vi "MT Detect MSK.vi"(5 "input complex waveform":T3={"t0"=0.0, "dt"=1.0, "Y"=[]} {"Y" format="%.3f"; "dt" format="%^.2e"; "t0" format="%.4f"}, 7 "MSK system parameters":T2={"differential encoding enable"=enum."enable", "samples per symbol (16)"=16}, 9 "synchronization parameters":T1 {"sync sequence" format="%.2f"}, 11 "error in (no error)":errorcluster, 12 "matched filter coefficients":dbl[](array[numeric]) format="%.2f", 13 "reset? (T)":bool=TRUE, 14 "flush buffers? (F)":bool) -> (6 "output bit stream":i8[](array[numeric]), 10 "sync found index (symbols)":dbl format="%.4f", 15 "error out":errorcluster)   [LabVIEW 2020, in "niDMT.lvlib"]
doc: "Demodulates an minimum-shift keying (MSK)-modulated complex baseband waveform and returns the demodulated bit stream. This VI attempts to remove carrier and phase offset by locking to the carrier signal."
uses:
  <vilib>/addons/Modulation/niDMT.lvlib
  <vilib>/addons/Modulation/Analog/controls/Complex Data Waveform.ctl
  <vilib>/Utility/error.llb/Error Cluster From Error Code.vi
  <vilib>/addons/Modulation/Digital/Support/Common/mod_Truncate FIR Filter (real).vi
  <vilib>/addons/Modulation/niAMT.lvlib
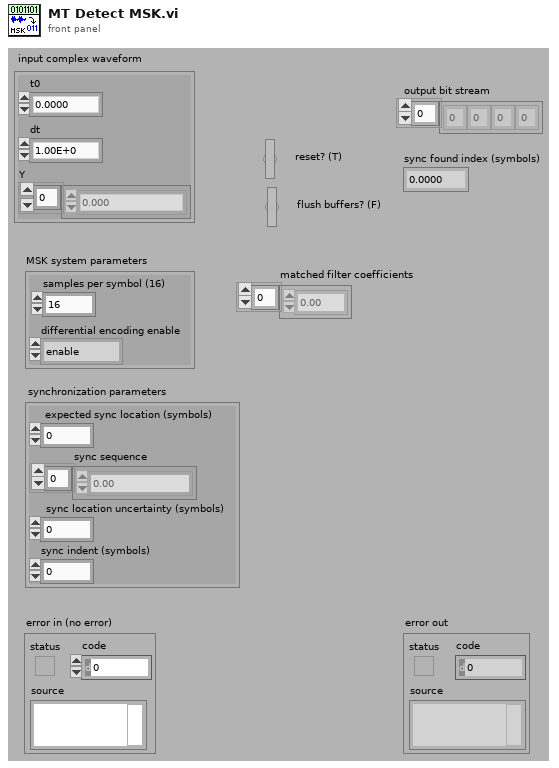
[diagram p1: front panel]
types:
  T1 = cluster{"expected sync location (symbols)":i32, "sync sequence":cdb[], "sync location uncertainty (symbols)":i32, "sync indent (symbols)":i32}
  T2 = cluster{"differential encoding enable":enum16{"disable", "enable"}, "samples per symbol (16)":i32}
  T3 = typedef "niAMT.lvlib/Complex Data Waveform.ctl" = cluster{"t0":dbl, "dt":dbl, "Y":cdb[]}
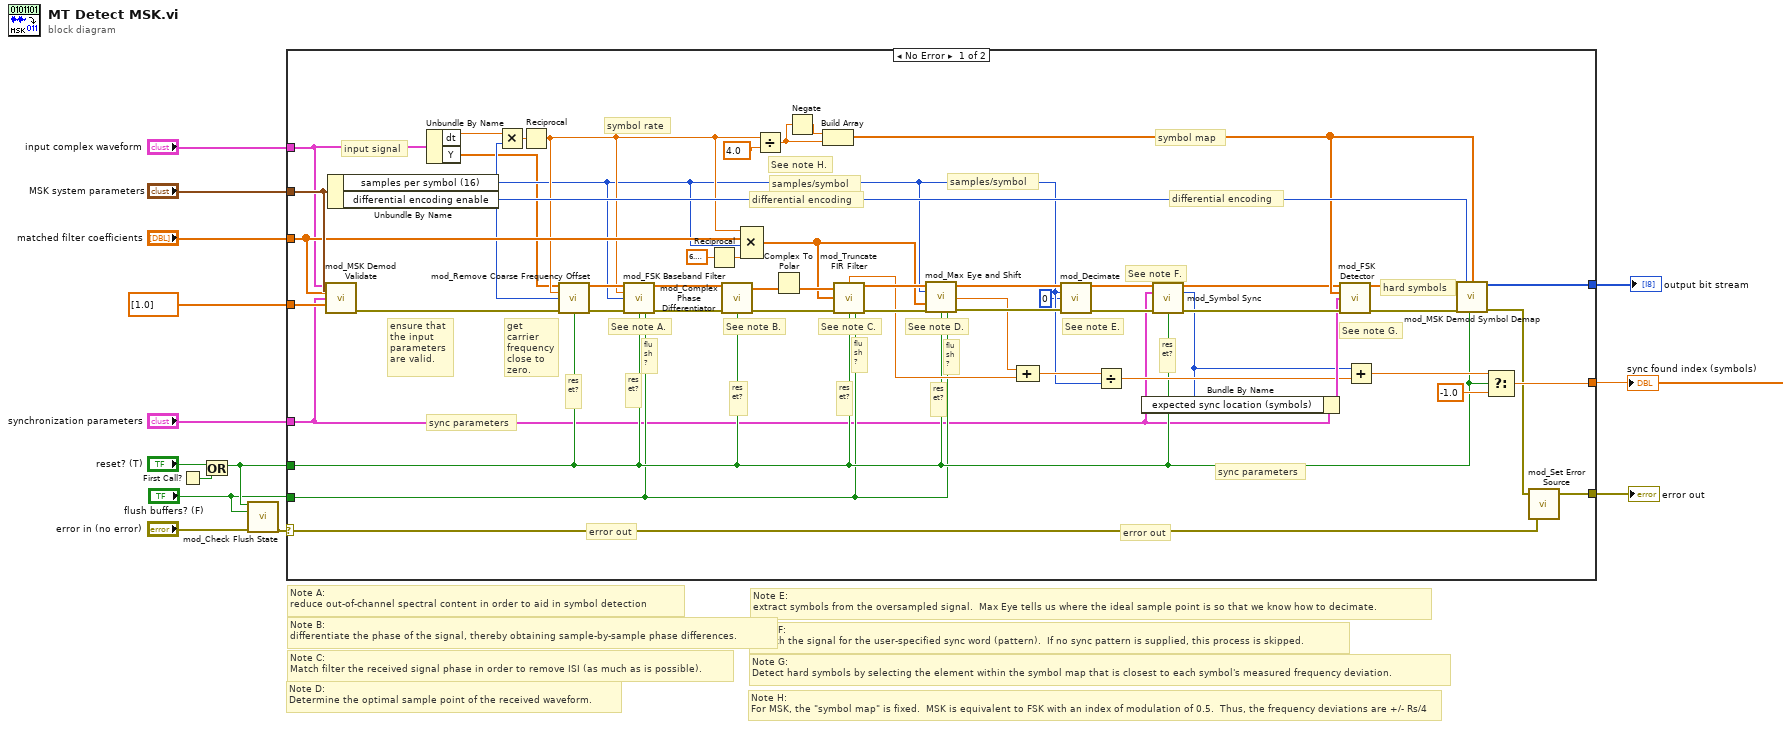
[diagram p0: block diagram]
diagram:
  # "Note H:\nFor MSK, the \"symbol map\" is fixed.  MSK is equivalent to FSK with an index of modulation of 0.5.  Thus, the frequency deviations are +/- Rs/4"
  # "Note A:\nreduce out-of-channel spectral content in order to aid in symbol detection"
  # "Note B:\ndifferentiate the phase of the signal, thereby obtaining sample-by-sample phase differences."
  # "Note C:\nMatch filter the received signal phase in order to remove ISI (as much as is possible)."
  # "Note D:\nDetermine the optimal sample point of the received waveform."
  # "Note E:\nextract symbols from the oversampled signal.  Max Eye tells us where the ideal sample point is so that we know how to decimate."
  # "Note F:\nSearch the signal for the user-specified sync word (pattern).  If no sync pattern is supplied, this process is skipped."
  # "Note G:\nDetect hard symbols by selecting the element within the symbol map that is closest to each symbol's measured frequency deviation."
  n1 = First Call?() -> (First Call?: T/F=w7:bool)
  n2 = Or(x="reset? (T)", y=w7) -> (x .or. y?=w3:bool)
  n3 = call <vilib>:"mod_Check Flush State.vi"("reset?"=w3, "flush buffers? (F)"="flush buffers? (F)", "error in (no error)"="error in (no error)") -> ("error out"=w4:errorcluster)  [unwired: 12 out]
  n4 = case shown="No Error" w4 {
    selector: w4 -> [w54 w67]
    tunnel: [w55 w67] -> w8
    tunnel: "synchronization parameters" -> [w15 _]
    tunnel: "matched filter coefficients" -> [w47 _]
    tunnel: "MSK system parameters" -> [w48 _]
    tunnel: dbl[] [1.0] ("pulse shaping filter coefficients") -> [w46 _]
    tunnel: [w33 _] -> w9
    tunnel: "input complex waveform" -> [w42 _]
    tunnel: [w60 _] -> w10
    tunnel: w3 -> [w27 _]
    tunnel: "flush buffers? (F)" -> [w16 _]
    frame No Error {
      # "See note H."
      # "flush?"
      # "flush?"
      # "flush?"
      # "reset?"
      # "sync parameters"
      # "sync parameters"
      # "error out"
      # "error out"
      # "reset?"
      # "reset?"
      # "reset?"
      # "reset?"
      # "reset?"
      # "detected bits"
      # "hard symbols"
      # "differential encoding"
      # "input signal"
      # "symbol rate"
      # "samples/symbol"
      # "samples/symbol"
      # "differential encoding"
      # "symbol rate"
      # "dt"
      # "symbol map"
      # "See note A."
      # "See note B."
      # "ensure that the input parameters are valid."
      # "get carrier frequency close to zero."
      # "See note D."
      # "See note E."
      # "See note C."
      # "See note F."
      # "See note G."
      n5 = call <vilib>:"mod_MSK Demod Validate.vi"("Input Complex Waveform"=w42, "MSK System Parameters"=w48, "Matched Filter Coefficients"=w47, "Synchronization Parameters"=w15, "Pulse Shaping Filter Coefficients"=w46) -> ("error out"=w49:errorcluster)  [unwired: 10 out]
      n6 = Unbundle By Name(w48) -> ("samples per symbol (16)"=w25:i32, "differential encoding enable"=w50:enum16{"disable", "enable"})
      n7 = Unbundle By Name(w42) -> ("dt"=w19:dbl, "Y"=w18:cdb[])
      n8 = Multiply(x=w19, y=w25) -> (x*y=w58:dbl)
      n9 = Reciprocal(x=w58) -> (1/x=w26:dbl)
      n10 = call <vilib>:"mod_Remove Coarse Frequency Offset.vi"("Signal In"=w18, "Symbol Rate, Hz"=w26, "Samples Per Symbol (16)"=w25, "error in (no error)"=w49, "Reset? (T)"=w27) -> ("Signal Out"=w29:cdb[], "error out"=w31:errorcluster)  [unwired: 9 out]
      n11 = call <vilib>:"mod_FSK Baseband Filter.vi"("Signal In"=w29, "Symbol Rate, Hz"=w26, "Samples Per Symbol (16)"=w25, "error in (no error)"=w31, "Reset? (T)"=w27, "flush buffers? (F)"=w16) -> ("Signal Out"=w28:cdb[], "error out"=w30:errorcluster)  [unwired: 8 in]
      n12 = Reciprocal(x=6.283185307179586) -> (1/x=w57:dbl)
      n13 = call <vilib>:"mod_Complex Phase Differentiator.vi"("Signal In"=w28, "error in (no error)"=w30, "Reset? (T)"=w27) -> ("Signal Out"=w43:cdb[], "error out"=w65:errorcluster)  [unwired: 11 out]
      n14 = Compound Arithmetic op=MULTIPLY(w26, w47, w25, w57) -> (w17:dbl[])
      n15 = Divide(x=w26, y=4.0) -> (x/y=w52:dbl)
      n16 = Complex To Polar(r * e^(i*theta)=w43) -> (theta=w59:dbl[])  [unwired: 1 out]
      n17 = Negate(x=w52) -> (-x=w51:dbl)
      n18 = Build Array(w51, w52) -> (w39:dbl[])
      n19 = call-poly <vilib>:"mod_Truncate FIR Filter.vi"("Signal In"=w59, "Filter Coefficients"=w17, "error in (no error)"=w65, "Reset? (T)"=w27, "flush buffers? (F)"=w16) -> ("Fractional Delay (samples)"=w37:dbl, "Signal Out"=w61:dbl[], "error out"=w64:errorcluster)  [unwired: 8 out]
      n20 = call <vilib>:"mod_Max Eye and Shift.vi"("Signal In"=w61, "Samples Per Symbol (16)"=w25, "matched filter coefficients"=w17, "error in (no error)"=w64, "Reset? (T)"=w27, "flush buffers? (F)"=w16) -> ("Signal Out"=w41:cdb[], "Optimal Offset (in Samples)"=w38:dbl, "error out"=w63:errorcluster)  [unwired: 7 out]
      n21 = Compound Arithmetic op=ADD(w38, w37) -> (w36:dbl)
      n22 = call <vilib>:"mod_Decimate.vi"("Signal In"=w41, "Samples Per Symbol (16)"=w25, "Offset"=0, "error in (no error)"=w63) -> ("Signal Out"=w40:cdb[], "error out"=w24:errorcluster)  [unwired: 1 in, 9 out]
      n23 = Divide(x=w36, y=w25) -> (x/y=w45:dbl)
      n24 = call <vilib>:"mod_Symbol Sync.vi"("Signal In"=w40, "Synchronization Parameters"=w15, "error in (no error)"=w24, "Reset? (T)"=w27) -> ("Signal Out"=w32:cdb[], "Sync Location (symbols)"=w44:i32, "error out"=w66:errorcluster)  [unwired: 9 out]
      n25 = Bundle By Name(cluster=w15, "expected sync location (symbols)"=w44) -> (w56:T1)
      n26 = call <vilib>:"mod_FSK Detector.vi"("Symbols"=w32, "Symbol Map"=w39, "Synchronization Parameters"=w56, "error in (no error)"=w66) -> ("Detected Symbols"=w23:dbl[], "error out"=w22:errorcluster)  [unwired: 1 in, 9 out]
      n27 = Add(x=w44, y=w45) -> (x+y=w35:dbl)
      n28 = call <vilib>:"mod_MSK Demod Symbol Demap.vi"("Symbols In"=w23, "Differential Encoding Enable"=w50, "Symbol Map"=w39, "error in (no error)"=w22, "Reset? (T)"=w27) -> ("Bits Out"=w60:i8[], "error out"=w21:errorcluster)  [unwired: 9 out]
      n29 = Select(t=w35, s=w27, f=-1.0) -> (s? t:f=w33:dbl)
      n30 = call <vilib>:"mod_Set Error Source.vi"("initial error in (no error)"=w54, "final error in (no error)"=w21) -> ("error out"=w55:errorcluster)  [unwired: 3 out]
    }
    frame Error {
    }
  }
  "error out" <- w8
  "sync found index (symbols)" <- w9
  "output bit stream" <- w10
